vi "KE622x -- Get Source Delay.vi"(0 "Resource In":refnum<visa-resource-name>, 1 "Check For SCPI Errors? (T)":bool=TRUE, 11 "error in (no error)":errorcluster) -> (4 "Resource Out (dupl)":refnum<visa-resource-name>, 8 "Source Delay (s)":dbl=0.001 min=0.001 max=1000.0 step=0.001 format="%.3f", 15 "error out":errorcluster)   [LabVIEW 2013, in "Keithly user program.lvlib"]
doc: "Returns the settling time (a.k.a. 'source delay') for all steps in a current sweep."
uses:
  Keithly user program.lvlib
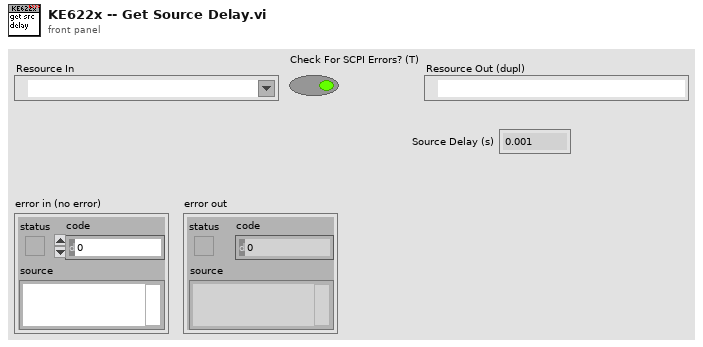
[diagram p1: front panel]
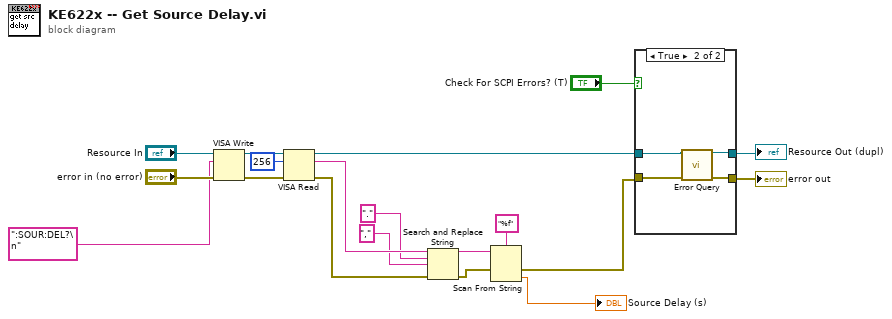
[diagram p0: block diagram]
diagram:
  n1 = VISA Write(VISA resource name="Resource In", write buffer=":SOUR:DEL?\n" ("format string"), error in (no error)="error in (no error)") -> (VISA resource name out=w13:refnum<visa-resource-name>, error out=w12:errorcluster)  [unwired: 1 out]
  n2 = VISA Read(VISA resource name=w13, byte count=u32 256, error in (no error)=w12) -> (VISA resource name out=w8:refnum<visa-resource-name>, read buffer=w3:string, error out=w4:errorcluster)  [unwired: 1 out]
  n3 = Search and Replace String(input string=w3, search string=".", replace string="," ("replace string (\"\")"), error in=w4) -> (result string=w6:string, error out=w5:errorcluster)  [unwired: 4 in, 2 out]
  n4 = Scan From String(format string="%f", input string=w6, error in=w5) -> (error out=w9:errorcluster, output 1=→"Source Delay (s)":dbl)  [unwired: 2 in, 2 out]
  n5 = case shown="True" "Check For SCPI Errors? (T)" {
    tunnel: w8 -> [w21 w25]
    tunnel: w9 -> [w20 w22]
    tunnel: [w20 w23] -> w15
    tunnel: [w21 w24] -> w16
    frame False {
    }
    frame True {
      n6 = call "Error Query.vi"("VISA Resource In"=w25, "error in (no error)"=w22) -> ("VISA Resource Out (dupl)"=w24:refnum<visa-resource-name>, "error out"=w23:errorcluster)  [unwired: 10 in, 2 out]
    }
  }
  "Resource Out (dupl)" <- w16
  "error out" <- w15
